vi "Global 3.vi"() -> ()   [LabVIEW 2021]
panel:
  in  "Boolean":bool
  in  "C":dbl
  in  "B":dbl
  in  "A":dbl
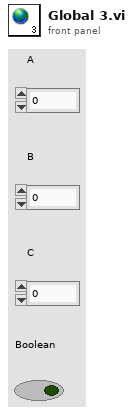
[diagram p1: front panel]
diagram:
